vi "Validate_Permission.vi"(8 "error in (no error)":errorcluster, 10 "file?":bool, 11 "Dest_NI_NIPath in":refnum<class "Dest_NI_NIPath.lvclass">) -> (0 "error out":errorcluster, 2 "valid?":bool, 3 "Dest_NI_NIPath out":refnum<class "Dest_NI_NIPath.lvclass">)   [LabVIEW 2020, in "Dest_NI_NIPath.lvclass"]
uses:
  <vilib>/AppBuilder/IB_Classes/Dest_NI_NIPath/Dest_NI_NIPath.lvclass
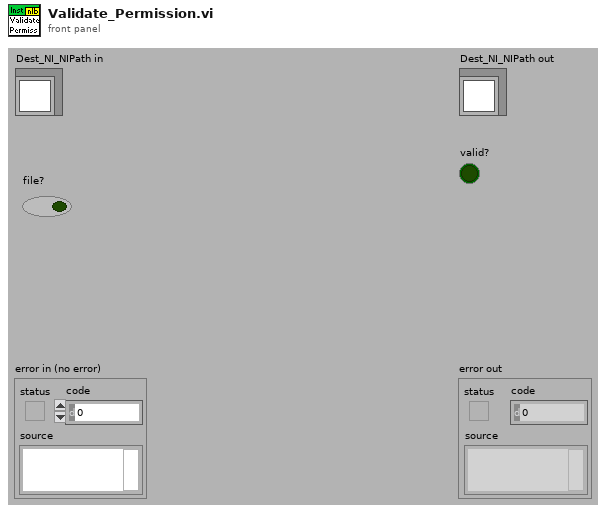
[diagram p1: front panel]
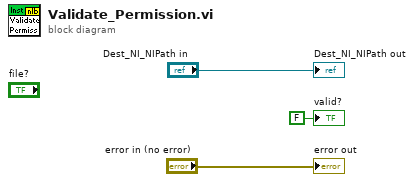
[diagram p0: block diagram]
diagram:
  "error out" <- "error in (no error)"
  "Dest_NI_NIPath out" <- "Dest_NI_NIPath in"
  "valid?" <- FALSE ("valid?")
